vi "Set-sequence-step.vi"(8 "error in (no error)":errorcluster, 10 "Sequence step in":i32, 11 "Object ref in":T1) -> (0 "error out":errorcluster, 2 "Sequence step":i32, 3 "Object ref out":T1)   [LabVIEW 2013, in "PowderDeposition.lvlib" / "PD-Main.lvclass"]
uses:
  PD-Main.lvclass
  Object-reference.ctl
  <vilib>/Utility/miscctls.llb/LVRowAndColumnTypeDef.ctl
  PD-Main.lvclass/PD-Main.ctl
  Read Motor sequences.vi
  Read Selected motor.vi
  Write Sequence index.vi
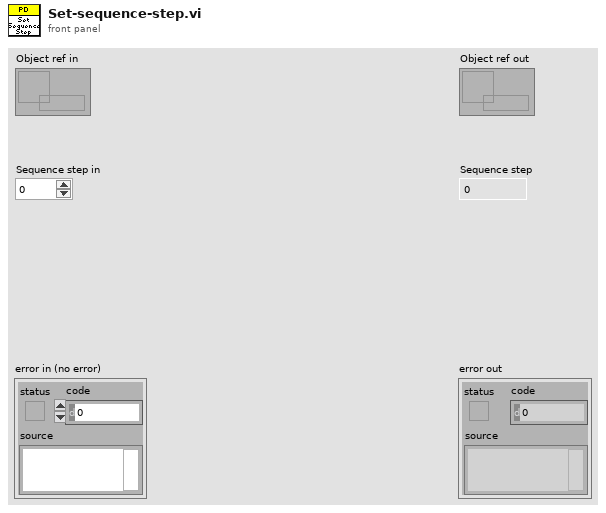
[diagram p1: front panel]
types:
  T1 = typedef "PowderDeposition.lvlib/PD-Main.lvclass/Object-reference.ctl" = refnum<data-value>
  T2 = typedef "LVRowAndColumnTypeDef.ctl" = cluster{"Row":i32, "Column":i32}
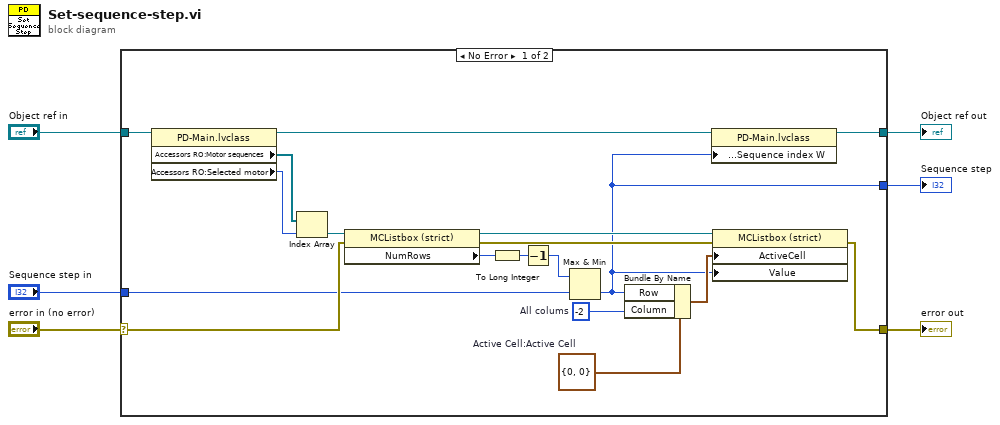
[diagram p0: block diagram]
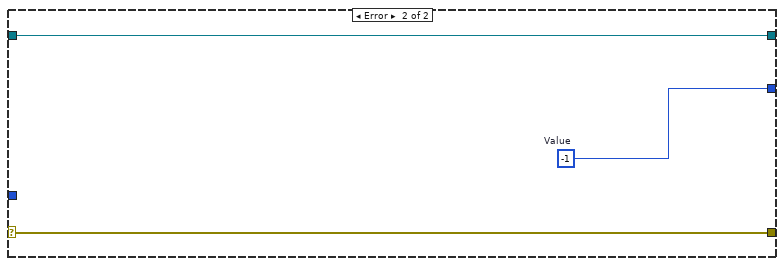
[diagram p2: hidden frame]
diagram:
  n1 = case shown="No Error" "error in (no error)" {
    selector: "error in (no error)" -> [w13 w27]
    tunnel: [w11 w27] -> w5
    tunnel: [w9 w26] -> w3
    tunnel: "Object ref in" -> [w24 w26]
    tunnel: [w8 w25] -> w2
    tunnel: "Sequence step in" -> [w10 _]
    frame No Error {
      w18 = -2  # All colums
      w19 = T2 {"Row"=0, "Column"=0}  # Active Cell:Active Cell
      n2 = property class="PD-Main.lvclass"(reference=w24) -> (reference out=w23:T1, "Accessors RO:Motor sequences"=w22:refnum<vi>[], "Accessors RO:Selected motor"=w7:i32)  [unwired: 1 in, 1 out]
      n3 = Index Array(array=w22, index=w7) -> (element=w21:refnum<vi>)
      n4 = property class="MCListbox (strict)"(reference=w21, error in=w13) -> (reference out=w15:refnum<vi>, error out=w12:errorcluster, "NumRows"=w14:u32)
      n5 = To Long Integer(number=w14) -> (32bit integer=w20:i32)
      n6 = Decrement(x=w20) -> (x-1=w16:i32)
      n7 = Max & Min(x=w16, y=w10) -> (min(x,y)=w8:i32)  [unwired: 1 out]
      n8 = Bundle By Name(cluster=w19, "Row"=w8, "Column"=w18) -> (w17:T2)
      n9 = property class="PD-Main.lvclass"(reference=w23, "Accessors/Modifiers:Sequence index W"=w8) -> (reference out=w9:T1)  [unwired: 1 in, 1 out]
      n10 = property class="MCListbox (strict)"(reference=w15, error in=w12, "ActiveCell"=w17, "Value"=w8) -> (error out=w11:errorcluster)  [unwired: 1 out]
    }
    frame Error {
      w25 = -1  # Value
    }
  }
  "error out" <- w5
  "Object ref out" <- w3
  "Sequence step" <- w2
